vi "Serialize - JSON.vi"(8 "error in":errorcluster, 11 "ePAS Data in":refnum<class "ePAS Data.lvclass">) -> (0 "error out":errorcluster, 2 "Serialized JSON":string, 3 "ePAS Data out":refnum<class "ePAS Data.lvclass">)   [LabVIEW 2018, in "ePAS Library.lvlib" / "ePAS Data.lvclass"]
uses:
  ePAS Data.lvclass
  ePAS Data.lvclass/ePAS Data.ctl
  reusable/PAS/Data/Main/PAS Data.lvclass
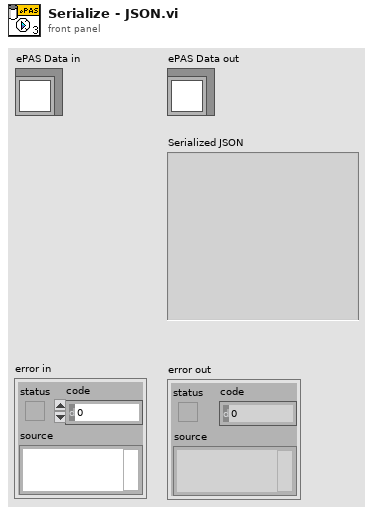
[diagram p1: front panel]
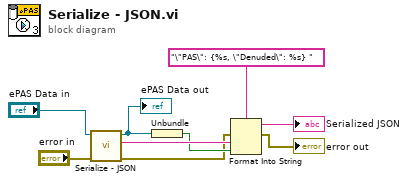
[diagram p0: block diagram]
diagram:
  n1 = call-parent "Serialize - JSON.vi"("error in"="error in", "PAS Data in"="ePAS Data in") -> ("error out"=w2:errorcluster, "Serialized JSON"=w6:string, "PAS Data out"=w7:refnum<class "ePAS Data.lvclass">)  [unwired: 7 in]
  "ePAS Data out" <- w7
  n2 = Unbundle(w7) -> (w4:bool)
  n3 = Format Into String(format string="\"PAS\": {%s, \"Denuded\": %s} ", error in=w2, w6, w4) -> (resulting string=→"Serialized JSON":string, error out=→"error out":errorcluster)  [unwired: 1 in]
